vi "命運+1000.vi"() -> ()   [LabVIEW 2014]
panel:
  in  "OK Button":bool
  in  "底色":u32(colorbox)=16768479
  # "系上終於有錢發獎勵金\n+1000"
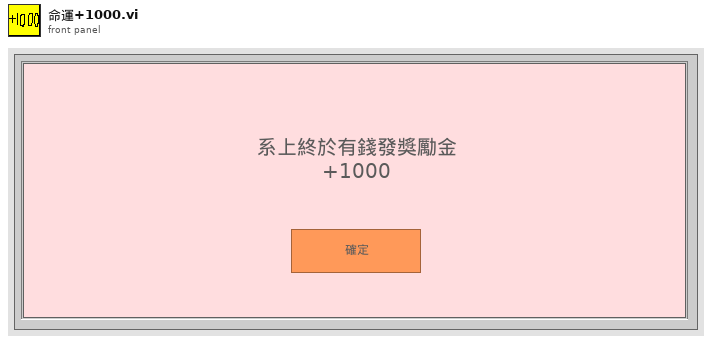
[diagram p1: front panel]
types:
  T1 = enum8{"Enabled", "Disabled", "Disabled and Grayed Out"}
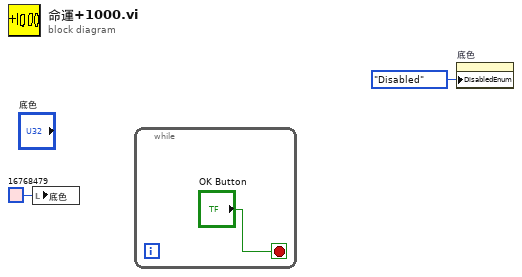
[diagram p0: block diagram]
diagram:
  n1 = local write "底色"(u32 16768479 ("底色")) -> ()
  n2 = while {
    stop <- "OK Button" stop-if-true
  }
  n3 = property on="底色" class="ColBox"("DisabledEnum"=T1."Disabled" ("Disabled")) -> ()  [unwired: 2 in, 2 out]
